vi "Joystick Control.vi"(9 "Enum":T1=enum."Run") -> (0 "Buttons Output Secondary":bool[](array[boolean]), 1 "Axis Output secondary":dbl[](array[numeric]), 2 "Button Output PJ":bool[](array[boolean]), 3 "Axis Output PJ":dbl[](array[numeric]), 4 "Axis Output PX":dbl[](array[numeric]), 5 "Buttons Output PX":bool[](array[boolean]))   [LabVIEW 2014]
uses:
  TypeDefs/SRE Enum.ctl
  <vilib>/Rock Robotics/WPI/Joystick/WPI_JoystickDeviceEnum.ctl
  Support Code/Robot Global Data.vi
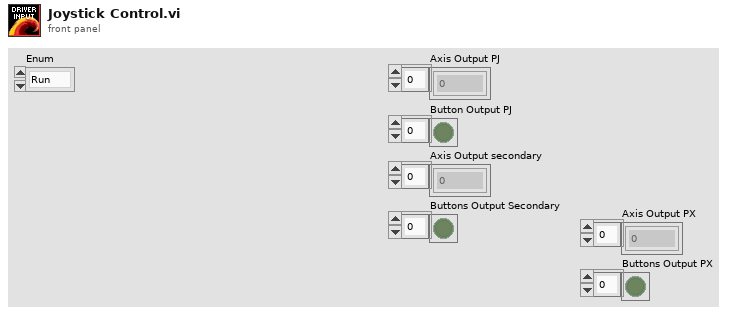
[diagram p1: front panel]
types:
  T1 = typedef "SRE Enum.ctl" = enum16{"Start", "Run", "End"}
  T2 = typedef "WPI_JoystickDeviceEnum.ctl" = enum16{"USB 0", "USB 1", "USB 2", "USB 3", "USB 4", "USB 5"}
  T3 = typedef "WPI_JoystickDevRef.ctl" = cluster{"Device":T2}
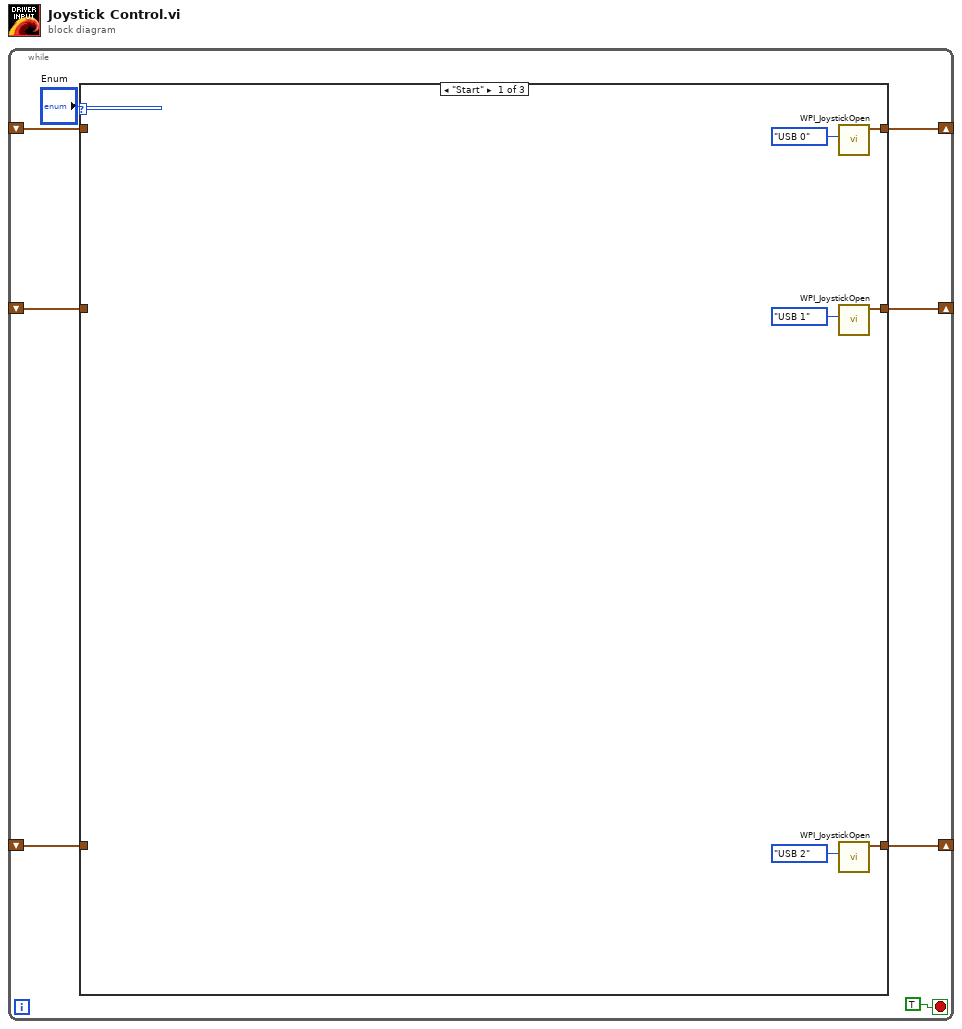
[diagram p0: block diagram]
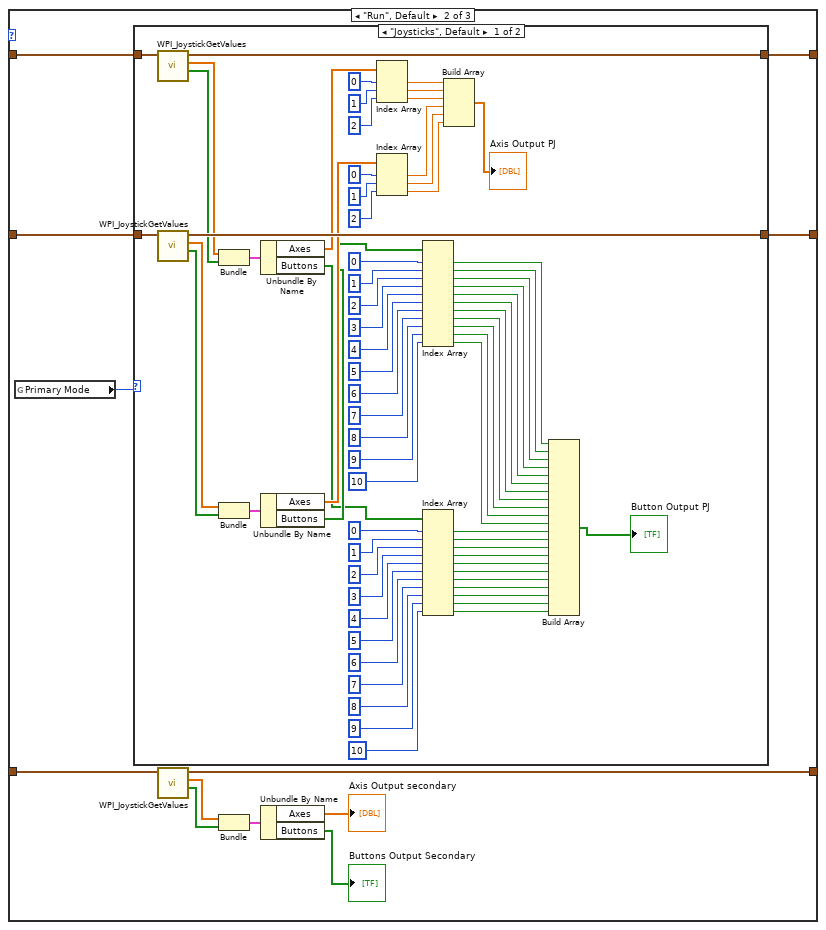
[diagram p2: hidden frame]
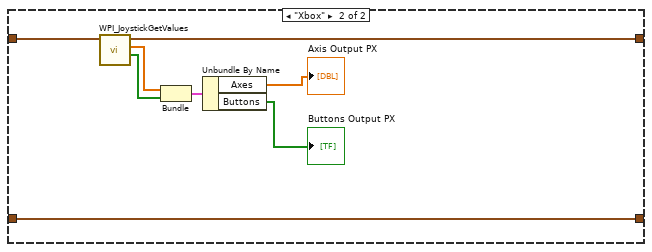
[diagram p3: hidden frame]
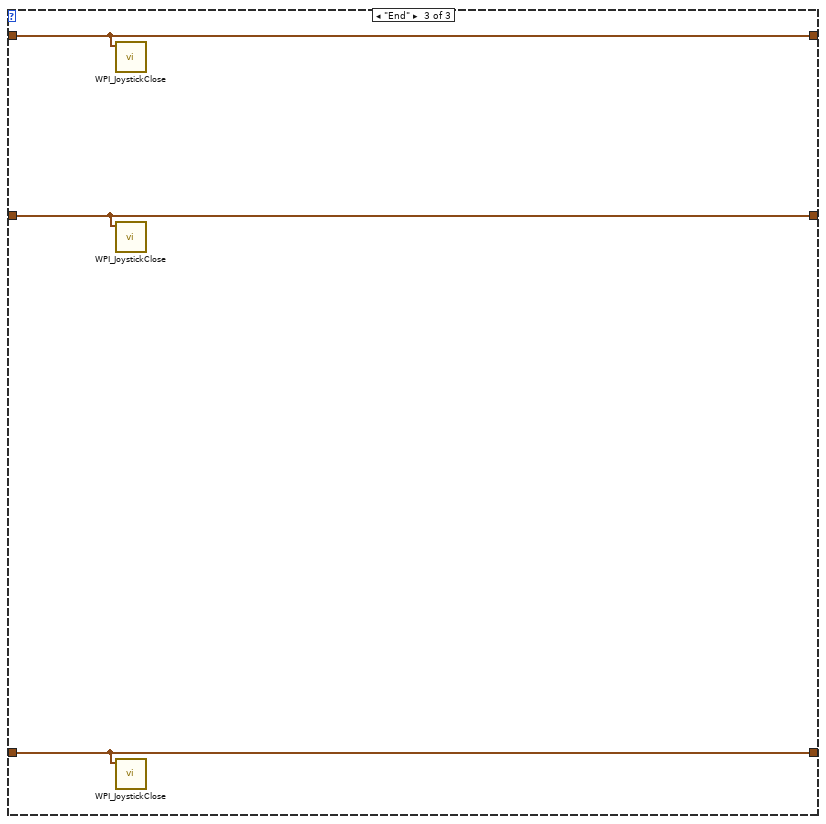
[diagram p4: hidden frame]
diagram:
  n1 = while {
    shift-right: [w7] -> _
    shift-left: _ -> [w4]
    shift-right: [w6] -> _
    shift-left: _ -> [w5]
    shift-right: [w2] -> _
    shift-left: _ -> [w1]
    stop <- TRUE stop-if-true
    n2 = case shown="\"Start\"" "Enum" {
      tunnel: [w14 w23 w108] -> w7
      tunnel: [w13 w25 w109] -> w6
      tunnel: w5 -> [_ w26 w109]
      tunnel: w4 -> [_ w24 w108]
      tunnel: [w9 w22 w107] -> w2
      tunnel: w1 -> [_ w21 w107]
      frame "Start" {
        n3 = call <vilib>:"WPI_JoystickOpen.vi"("JoystickDevice"=WPI_JoystickDeviceEnum."USB 0") -> ("JoystickDevRef"=w14:T3)  [unwired: 10 in]
        n4 = call <vilib>:"WPI_JoystickOpen.vi"("JoystickDevice"=WPI_JoystickDeviceEnum."USB 1") -> ("JoystickDevRef"=w13:T3)  [unwired: 10 in]
        n5 = call <vilib>:"WPI_JoystickOpen.vi"("JoystickDevice"=WPI_JoystickDeviceEnum."USB 2") -> ("JoystickDevRef"=w9:T3)  [unwired: 10 in]
      }
      frame "Run", Default {
        n6 = global read "Robot Global Data.vi" "Primary Mode"() -> (w15:enum16{"Joysticks", "Xbox"})
        n7 = case shown="\"Joysticks\", Default" w15 {
          tunnel: w26 -> [w98 w103]
          tunnel: [w97 w103] -> w25
          tunnel: w24 -> [w96 w102]
          tunnel: [w95 w101] -> w23
          frame "Joysticks", Default {
            n8 = call <vilib>:"WPI_JoystickGetValues.vi"("JoystickDevRef"=w96) -> ("Buttons"=w93:bool[], "Axes"=w94:dbl[], "JoystickDevRef"=w95:T3)  [unwired: 6 in, 2 out]
            n9 = call <vilib>:"WPI_JoystickGetValues.vi"("JoystickDevRef"=w98) -> ("Buttons"=w91:bool[], "Axes"=w92:dbl[], "JoystickDevRef"=w97:T3)  [unwired: 6 in, 2 out]
            n10 = Bundle("Axes"=w94, "Buttons"=w93) -> (w90:cluster{"Axes":dbl[], "Buttons":bool[]})  [unwired: 1 in]
            n11 = Bundle("Axes"=w92, "Buttons"=w91) -> (w89:cluster{"Axes":dbl[], "Buttons":bool[]})  [unwired: 1 in]
            n12 = Unbundle By Name(w90) -> ("Axes"=w88:dbl[], "Buttons"=w29:bool[])
            n13 = Unbundle By Name(w89) -> ("Axes"=w87:dbl[], "Buttons"=w30:bool[])
            n14 = Index Array(array=w88, index #1=0 ("index"), index #2=1 ("index"), index #3=2 ("index")) -> (element #1=w80:dbl, element #2=w79:dbl, element #3=w78:dbl)
            n15 = Index Array(array=w87, index #1=0 ("index"), index #2=1 ("index"), index #3=2 ("index")) -> (element #1=w77:dbl, element #2=w76:dbl, element #3=w75:dbl)
            n16 = Index Array(array=w30, index #1=0 ("index"), index #2=1 ("index"), index #3=2 ("index"), index #4=3 ("index"), index #5=4 ("index"), index #6=5 ("index"), index #7=6 ("index"), index #8=7 ("index"), index #9=8 ("index"), index #10=9 ("index"), index #11=10 ("index")) -> (element #1=w74:bool, element #2=w73:bool, element #3=w72:bool, element #4=w60:bool, element #5=w59:bool, element #6=w58:bool, element #7=w57:bool, element #8=w56:bool, element #9=w55:bool, element #10=w54:bool, element #11=w53:bool)
            n17 = Index Array(array=w29, index #1=0 ("index"), index #2=1 ("index"), index #3=2 ("index"), index #4=3 ("index"), index #5=4 ("index"), index #6=5 ("index"), index #7=6 ("index"), index #8=7 ("index"), index #9=8 ("index"), index #10=9 ("index"), index #11=10 ("index")) -> (element #1=w41:bool, element #2=w40:bool, element #3=w39:bool, element #4=w38:bool, element #5=w37:bool, element #6=w36:bool, element #7=w35:bool, element #8=w34:bool, element #9=w33:bool, element #10=w32:bool, element #11=w31:bool)
            n18 = Build Array(w80, w79, w78, w77, w76, w75) -> (→"Axis Output PJ":dbl[])
            n19 = Build Array(w74, w73, w72, w60, w59, w58, w57, w56, w55, w54, w53, w41, w40, w39, w38, w37, w36, w35, w34, w33, w32, w31) -> (→"Button Output PJ":bool[])
          }
          frame "Xbox" {
            n20 = call <vilib>:"WPI_JoystickGetValues.vi"("JoystickDevRef"=w102) -> ("Buttons"=w104:bool[], "Axes"=w105:dbl[], "JoystickDevRef"=w101:T3)  [unwired: 6 in, 2 out]
            n21 = Bundle("Axes"=w105, "Buttons"=w104) -> (w106:cluster{"Axes":dbl[], "Buttons":bool[]})  [unwired: 1 in]
            n22 = Unbundle By Name(w106) -> ("Axes"=→"Axis Output PX":dbl[], "Buttons"=→"Buttons Output PX":bool[])
          }
        }
        n23 = call <vilib>:"WPI_JoystickGetValues.vi"("JoystickDevRef"=w21) -> ("Buttons"=w18:bool[], "Axes"=w19:dbl[], "JoystickDevRef"=w22:T3)  [unwired: 6 in, 2 out]
        n24 = Bundle("Axes"=w19, "Buttons"=w18) -> (w20:cluster{"Axes":dbl[], "Buttons":bool[]})  [unwired: 1 in]
        n25 = Unbundle By Name(w20) -> ("Axes"=→"Axis Output secondary":dbl[], "Buttons"=→"Buttons Output Secondary":bool[])
      }
      frame "End" {
        n26 = call <vilib>:"WPI_JoystickClose.vi"("JoystickDevRef"=w108) -> ()  [unwired: 11 in]
        n27 = call <vilib>:"WPI_JoystickClose.vi"("JoystickDevRef"=w109) -> ()  [unwired: 11 in]
        n28 = call <vilib>:"WPI_JoystickClose.vi"("JoystickDevRef"=w107) -> ()  [unwired: 11 in]
      }
    }
  }
